vi "Package Data.vi"(8 "error in":errorcluster, 10 "DataIn":string, 11 "MC Data in":refnum<class "MC Data.lvclass">) -> (0 "error out":errorcluster, 3 "MC Data out":refnum<class "MC Data.lvclass">)   [LabVIEW 2015, in "Alicat Lib.lvlib" / "MC Data.lvclass"]
uses:
  MC Data.lvclass
  MC Data.lvclass/MC Data.ctl
  <vilib>/MSR Consulting, LLC/General Reuse/General/Atmospheric/Atmospheric Constants.vi
  <vilib>/MSR Consulting, LLC/General Reuse/Data/Write measTime.vi
  <vilib>/MSR Consulting, LLC/General Reuse/General/Atmospheric/Atmospheric Library.lvlib
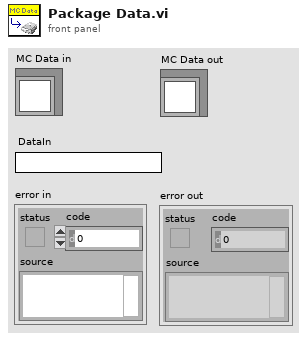
[diagram p1: front panel]
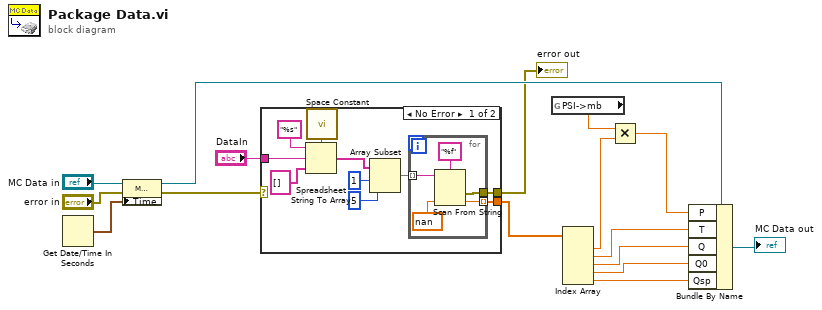
[diagram p0: block diagram]
diagram:
  n1 = Get Date/Time In Seconds() -> (seconds since 1Jan1904=w1:timestamp)
  n2 = property class="MC Data"(reference="MC Data in", error in="error in", "Time"=w1) -> (reference out=w5:refnum<class "MC Data.lvclass">, error out=w3:errorcluster)
  n3 = case shown="No Error" w3 {
    selector: w3 -> [_ w32]
    tunnel: "DataIn" -> [w23 _]
    tunnel: [w18 _] -> w8
    tunnel: [w22 w32] -> w2
    frame No Error {
      n4 = call <vilib>:"Space Constant.vi"() -> ("String"=w25:string)
      n5 = Spreadsheet String To Array(delimiter (Tab)=w25, format string="%s", spreadsheet string=w23, array type (2D Dbl)=string[] []) -> (array=w21:string[])
      n6 = Array Subset(array=w21, index=1, length=5) -> (w19:string[])
      n7 = for {
        tunnel: w19 -> [w27] mode=indexing
        tunnel: [w29] -> w18 mode=indexing
        tunnel: [w28] -> w22
        n8 = Scan From String(format string="%f", input string=w27, default 1=sgl nan ("default value 1")) -> (error out=w28:errorcluster, output 1=w29:sgl)  [unwired: 2 in, 2 out]
      }
    }
    frame Error {
    }
  }
  "error out" <- w2
  n9 = global read "Atmospheric Constants.vi" "PSI->mb"() -> (w9:sgl)
  n10 = Index Array(array=w8) -> (element #1=w14:sgl, element #2=w13:sgl, element #3=w12:sgl, element #4=w11:sgl, element #5=w10:sgl)  [unwired: 5 in]
  n11 = Multiply(x=w9, y=w14) -> (x*y=w15:sgl)
  n12 = Bundle By Name(cluster=w5, "P"=w15, "T"=w13, "Q"=w12, "Q0"=w11, "Qsp"=w10) -> (→"MC Data out":refnum<class "MC Data.lvclass">)
